vi "Main Tree _ Click Event Pharse(tag).vi"(8 "error in":errorcluster caption="错误输入", 10 "tag in":string, 11 "Ref.Tree Ref":refnum<vi>) -> (0 "error out":errorcluster caption="错误输出", 1 "cmd?":bool, 2 "LocalData":variant, 3 "LocalEvent":string)   [LabVIEW 2016]
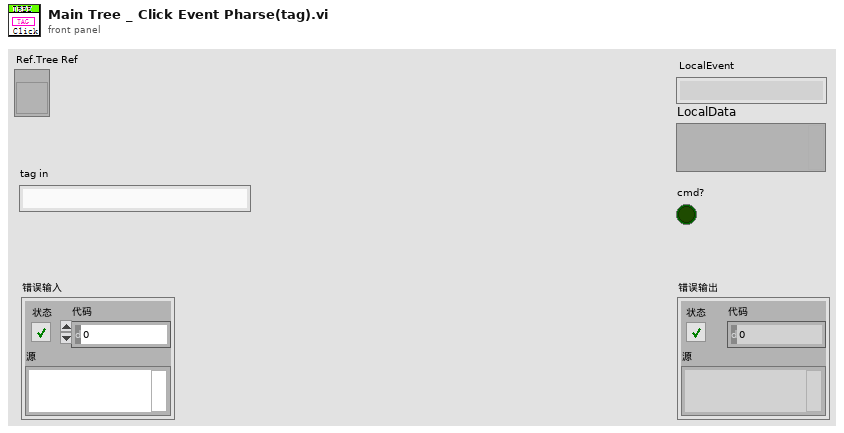
[diagram p1: front panel]
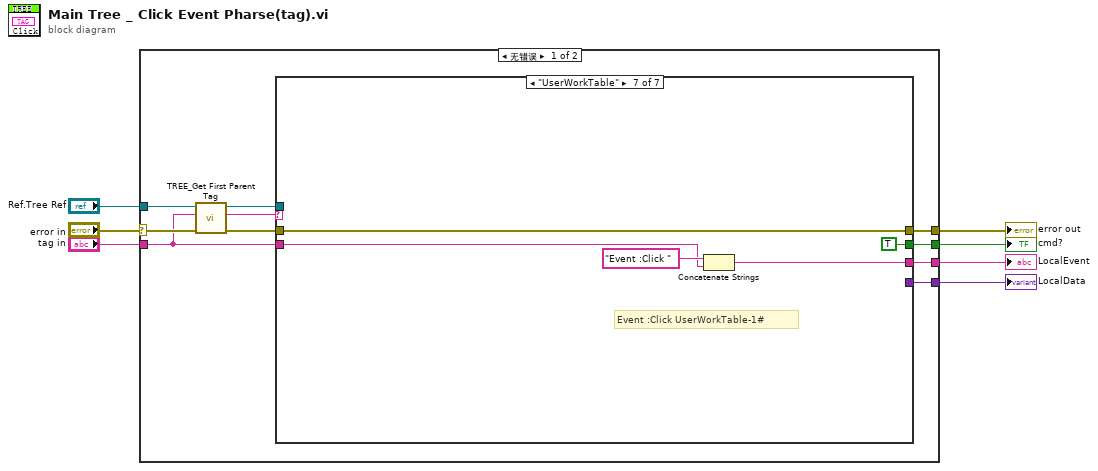
[diagram p0: block diagram]
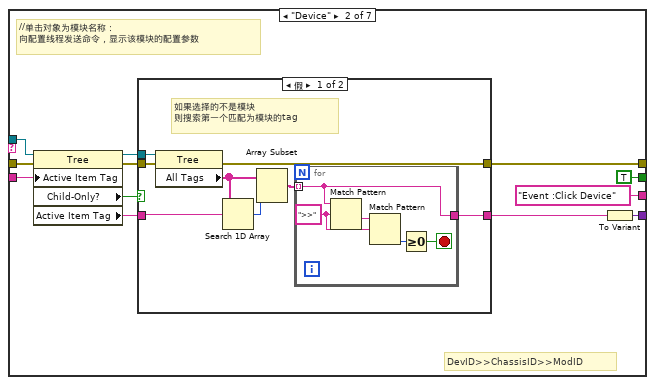
[diagram p3: hidden frame]
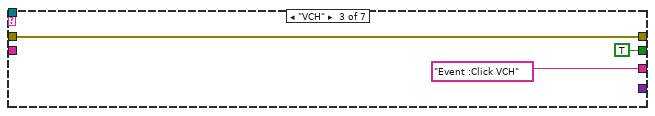
[diagram p5: hidden frame]
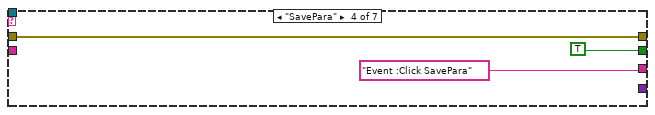
[diagram p6: hidden frame]
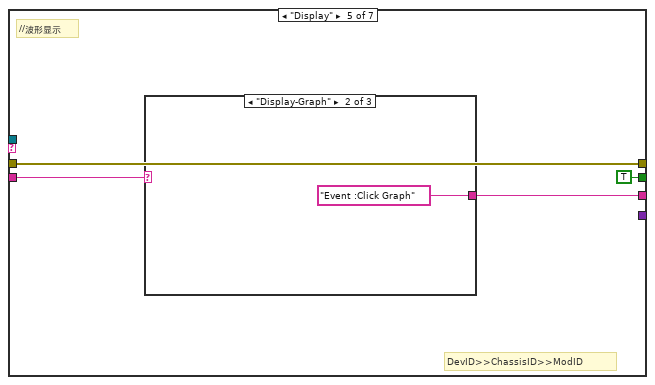
[diagram p7: hidden frame]
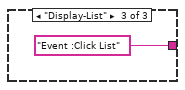
[diagram p9: hidden frame]
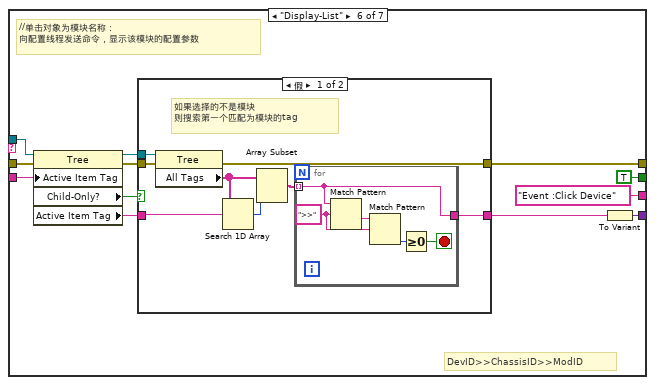
[diagram p10: hidden frame]
diagram:
  n1 = case shown="无错误" "error in" {
    selector: "error in" -> [w12 w90]
    tunnel: [w15 w90] -> w6
    tunnel: "Ref.Tree Ref" -> [w13 _]
    tunnel: "tag in" -> [w8 _]
    tunnel: [w17 _] -> w3
    tunnel: [w16 _] -> w2
    tunnel: [w14 _] -> w1
    frame No Error {
      n2 = call "TREE_Get First Parent Tag.vi"("error in"=w12, "tag in"=w8, "Tree Ref"=w13) -> ("error out"=w11:errorcluster, "tag out"=w9:string, "Tree Ref"=w10:refnum<vi>)  [unwired: 6 in]
      n3 = case shown="\"UserWorkTable\"" w9 {
        tunnel: [_ "Event :Click Device" ("正则表达式") "Event :Click VCH" ("正则表达式") "Event :Click SavePara" ("正则表达式") w52 "Event :Click Device" ("正则表达式") w85] -> w14
        tunnel: w11 -> [w18 w30 w48 w51 w54 w69 w89]
        tunnel: w10 -> [_ w29 _ _ _ w68 _]
        tunnel: [_ TRUE ("Child-Only?") TRUE ("Child-Only?") TRUE ("Child-Only?") TRUE ("Child-Only?") TRUE ("Child-Only?") TRUE ("Child-Only?")] -> w17
        tunnel: w8 -> [_ w28 _ _ w53 w67 w86]
        tunnel: [w18 w19 w48 w51 w54 w58 w89] -> w15
        tunnel: [_ w25 _ _ _ w64 _] -> w16
        frame Default {
        }
        frame "Device" {
          # "DevID>>ChassisID>>ModID"
          # "//单击对象为模块名称：\n向配置线程发送命令，显示该模块的配置参数"
          n4 = property class="Tree"(reference=w29, error in=w30, "Active Item Tag"=w28) -> (reference out=w21:refnum<vi>, error out=w20:errorcluster, "Child-Only?"=w24:bool, "Active Item Tag"=w22:string)
          n5 = case shown="假" w24 {
            tunnel: [w32 w45] -> w23
            tunnel: w22 -> [w36 w45]
            tunnel: w21 -> [w38 _]
            tunnel: w20 -> [w37 w44]
            tunnel: [w31 w44] -> w19
            frame False {
              # "如果选择的不是模块\n则搜索第一个匹配为模块的tag"
              n6 = property class="Tree"(reference=w38, error in=w37) -> (error out=w31:errorcluster, "All Tags"=w35:string[])  [unwired: 1 out]
              n7 = Search 1D Array(1D array=w35, element=w36) -> (index of element=w34:i32)  [unwired: 1 in]
              n8 = Array Subset(array=w35, index=w34) -> (w33:string[])  [unwired: 1 in]
              n9 = for {
                tunnel: w33 -> [w39] mode=indexing
                tunnel: [w39] -> w32
                stop <- w40 stop-if-true
                w42 = ">>" ("正则表达式")
                n10 = Match Pattern(string=w39, regular expression=w42) -> (after substring=w43:string)  [unwired: 1 in, 3 out]
                n11 = Match Pattern(string=w43, regular expression=w42) -> (offset past match=w41:i32)  [unwired: 1 in, 3 out]
                n12 = Greater Or Equal To 0?(x=w41) -> (x >= 0?=w40:bool)
              }
            }
            frame True {
            }
          }
          n13 = To Variant(anything=w23) -> (Variant=w25:variant)
        }
        frame "VCH" {
        }
        frame "SavePara" {
        }
        frame "Display" {
          # "DevID>>ChassisID>>ModID"
          # "//波形显示"
          n14 = case shown="\"Display-Graph\"" w53 {
            tunnel: [_ "Event :Click Graph" ("正则表达式") "Event :Click List" ("正则表达式")] -> w52
            frame "False", Default {
            }
            frame "Display-Graph" {
            }
            frame "Display-List" {
            }
          }
        }
        frame "Display-List" {
          # "DevID>>ChassisID>>ModID"
          # "//单击对象为模块名称：\n向配置线程发送命令，显示该模块的配置参数"
          n15 = property class="Tree"(reference=w68, error in=w69, "Active Item Tag"=w67) -> (reference out=w60:refnum<vi>, error out=w59:errorcluster, "Child-Only?"=w63:bool, "Active Item Tag"=w61:string)
          n16 = case shown="假" w63 {
            tunnel: [w71 w84] -> w62
            tunnel: w61 -> [w75 w84]
            tunnel: w60 -> [w77 _]
            tunnel: w59 -> [w76 w83]
            tunnel: [w70 w83] -> w58
            frame False {
              # "如果选择的不是模块\n则搜索第一个匹配为模块的tag"
              n17 = property class="Tree"(reference=w77, error in=w76) -> (error out=w70:errorcluster, "All Tags"=w74:string[])  [unwired: 1 out]
              n18 = Search 1D Array(1D array=w74, element=w75) -> (index of element=w73:i32)  [unwired: 1 in]
              n19 = Array Subset(array=w74, index=w73) -> (w72:string[])  [unwired: 1 in]
              n20 = for {
                tunnel: w72 -> [w78] mode=indexing
                tunnel: [w78] -> w71
                stop <- w79 stop-if-true
                w81 = ">>" ("正则表达式")
                n21 = Match Pattern(string=w78, regular expression=w81) -> (after substring=w82:string)  [unwired: 1 in, 3 out]
                n22 = Match Pattern(string=w82, regular expression=w81) -> (offset past match=w80:i32)  [unwired: 1 in, 3 out]
                n23 = Greater Or Equal To 0?(x=w80) -> (x >= 0?=w79:bool)
              }
            }
            frame True {
            }
          }
          n24 = To Variant(anything=w62) -> (Variant=w64:variant)
        }
        frame "UserWorkTable" {
          # "Event :Click UserWorkTable-1#"
          n25 = Concatenate Strings("Event :Click " ("正则表达式"), w86) -> (w85:string)
        }
      }
    }
    frame Error {
    }
  }
  "error out" <- w6
  "LocalEvent" <- w1
  "LocalData" <- w2
  "cmd?" <- w3
